vi "Write PassObserverRole.vi"(8 "error in (no error)":errorcluster, 10 "PassObserverRole":refnum<class "PassObserverRole.lvclass">, 11 "Rolebook in":refnum<class "Rolebook.lvclass">) -> (0 "error out":errorcluster, 3 "Rolebook out":refnum<class "Rolebook.lvclass">)   [LabVIEW 2018, in "Rolebook.lvclass"]
uses:
  Rolebook.lvclass
  PassObserverRole_class/PassObserverRole.lvclass
  Rolebook.lvclass/Rolebook.ctl
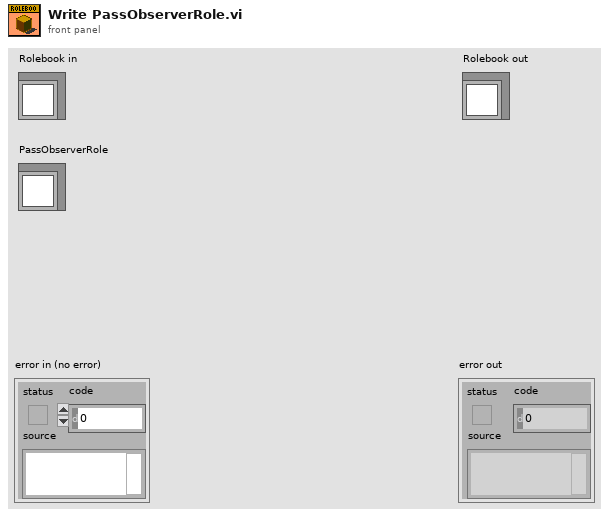
[diagram p1: front panel]
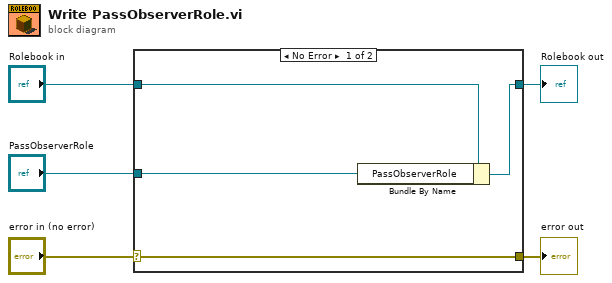
[diagram p0: block diagram]
diagram:
  n1 = case shown="No Error" "error in (no error)" {
    selector: "error in (no error)" -> [w9 w10]
    tunnel: [w9 w10] -> w4
    tunnel: [w7 w11] -> w2
    tunnel: "Rolebook in" -> [w8 w11]
    tunnel: "PassObserverRole" -> [w6 _]
    frame No Error {
      n2 = Bundle By Name(cluster=w8, "PassObserverRole"=w6) -> (w7:refnum<class "Rolebook.lvclass">)
    }
    frame Error {
    }
  }
  "error out" <- w4
  "Rolebook out" <- w2
